vi "Lockin.getDAQPublicEvents.vi"(8 "error in (no error)":errorcluster, 11 "Instrument.Lockin in":refnum<class "Instrument.Lockin.lvclass">) -> (0 "error out":errorcluster, 1 "DAQ SMO Public Events":T2, 2 "DAQ Public Events":T1, 3 "Instrument.Lockin out":refnum<class "Instrument.Lockin.lvclass">)   [LabVIEW 2019, in "Instrument.Lockin.lvlib" / "Instrument.Lockin.lvclass"]
uses:
  Instrument.Lockin.lvclass
  <vilib>/JKI/JKI SMO/SMO/Typedefs/Public Events.ctl
  <vilib>/JKI/JKI SMO/SMO/Typedefs/SMOState --Enum.ctl
  <vilib>/JKI/JKI SMO/SMO/Typedefs/Reserve State--Enum.ctl
  Instrument.DAQ/Typedefs/PublicEvents--Cluster.ctl
  Instrument.DAQ/Typedefs/PublicEvents--DAQ.getAIChannels.ctl
  Instrument.DAQ/Typedefs/AI.Channel--Cluster--Array.ctl
  Instrument.DAQ/Typedefs/AI.Channel--Cluster.ctl
  Instrument.DAQ/Typedefs/PublicEvents--DAQ.getAOChannels.ctl
  Instrument.DAQ/Typedefs/AO.Channel--Cluster--Array.ctl
  Instrument.DAQ/Typedefs/AO.Channel--Cluster.ctl
  Instrument.DAQ/Typedefs/AO.Channel.Function--Enum.ctl
  Instrument.DAQ/Typedefs/PublicEvents--DAQ.getREFChannels.ctl
  Instrument.DAQ/Typedefs/REF.Channel--Cluster--Array.ctl
  Instrument.DAQ/Typedefs/REF.Channel--Cluster.ctl
  Instrument.DAQ/Typedefs/PublicEvents--DAQ.getWaveforms.ctl
  Instrument.DAQ/Typedefs/PublicEvents--DAQ.getResults.ctl
  Instrument.DAQ/Typedefs/Results--Cluster.ctl
  Instrument.DAQ/Typedefs/PublicEvents--DAQ.getSweepWaveforms.ctl
  Instrument.DAQ/Typedefs/PublicEvents--DAQ.getCalibration.ctl
  Instrument.DAQ/Typedefs/DAQ.Calibration--Cluster--Array.ctl
  Instrument.DAQ/Typedefs/DAQ.Calibration--Cluster.ctl
  Instrument.DAQ/Typedefs/PublicEvents--DAQ.getDAQState.ctl
  Instrument.DAQ/Typedefs/Status--enum.ctl
  Instrument.DAQ/Typedefs/PublicEvents--DAQ.getDAQconfig.ctl
  Instrument.DAQ/Typedefs/DAQ.Configuration--Cluster--Array.ctl
  Instrument.DAQ/Typedefs/DAQ.Configuration--Cluster.ctl
  Instrument.DAQ/Typedefs/DAQ.Config.AO.Range--enum.ctl
  Instrument.DAQ/Typedefs/DAQ.TerminalConfiguration--ring.ctl
  Instrument.DAQ/Typedefs/DAQ.Config.AI.Range--enum.ctl
  Instrument.DAQ/Typedefs/DAQ.Config.AI.Coupling--enum.ctl
  Instrument.DAQ/Typedefs/PublicEvents--DAQ.getInputGain.ctl
  Instrument.DAQ/Typedefs/Channel.Gain--Cluster--Array.ctl
  Instrument.DAQ/Typedefs/Channel.Gain--Cluster.ctl
  Instrument.DAQ/Typedefs/PublicEvents--DAQ.getOutputGain.ctl
  Instrument.DAQ/Typedefs/PublicEvents--DAQ.getInputOffset.ctl
  Instrument.DAQ/Typedefs/PublicEvents--DAQ.getSampling.ctl
  Instrument.DAQ/Typedefs/DAQ.Sampling--Cluster.ctl
  Instrument.DAQ/Typedefs/DAQ.Sampling.Sampling--Cluster.ctl
  Instrument.DAQ/Typedefs/DAQ.Sampling.Fs Mode--enum.ctl
  Instrument.DAQ/Typedefs/PublicEvents--DAQ.getSweepChannels.ctl
  Instrument.DAQ/Typedefs/Sweep.Configuration--Cluster.ctl
  Instrument.DAQ/Typedefs/Sweep.Channel--Cluster--Array.ctl
  Instrument.DAQ/Typedefs/Sweep.Channel--Cluster.ctl
  Instrument.DAQ/Typedefs/Sweep.Pattern--Enum.ctl
  Instrument.DAQ/Typedefs/PublicEvents--DAQ.getDeviceIDN.ctl
  Instrument.DAQ/Typedefs/DeviceInfo--Cluster.ctl
  <vilib>/JKI/JKI SMO/SMO/SMO.lvclass/SMO.ctl
  <vilib>/JKI/JKI SMO/SMO/Private/ReftoDVR--SMO.vi
  Instrument.DAQ/Instrument.DAQ.lvclass
  C:/Program Files/National Instruments/LabVIEW 2019/vi.lib/JKI/JKI SMO/SMO/SMO.lvclass
  <vilib>/JKI/JKI SMO/SMO/SMO.lvclass
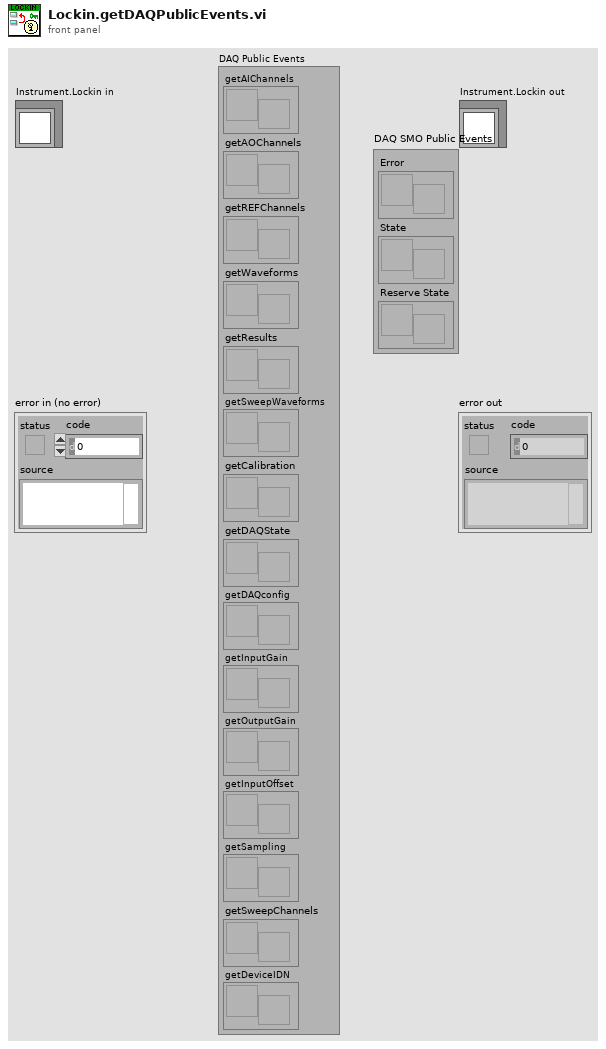
[diagram p1: front panel]
types:
  T1 = typedef "Instrument.Lockin.lvlib/Instrument.DAQ.lvclass/PublicEvents--Cluster.ctl" = cluster{"getAIChannels":refnum<user-event>, "getAOChannels":refnum<user-event>, "getREFChannels":refnum<user-event>, "getWaveforms":refnum<user-event>, "getResults":refnum<user-event>, "getSweepWaveforms":refnum<user-event>, "getCalibration":refnum<user-event>, "getDAQState":refnum<user-event>, "getDAQconfig":refnum<user-event>, "getInputGain":refnum<user-event>, "getOutputGain":refnum<user-event>, "getInputOffset":refnum<user-event>, "getSampling":refnum<user-event>, "getSweepChannels":refnum<user-event>, "getDeviceIDN":refnum<user-event>}
  T2 = typedef "SMO.lvclass/Public Events.ctl" = cluster{"Error":refnum<user-event>, "State":refnum<user-event>, "Reserve State":refnum<user-event>}
  T3 = typedef "Instrument.Lockin.lvlib/Instrument.Lockin.lvclass/Lockin.Dependencies--Cluster.ctl" = cluster{"Instrument.DAQ":refnum<class "Instrument.DAQ.lvclass">}
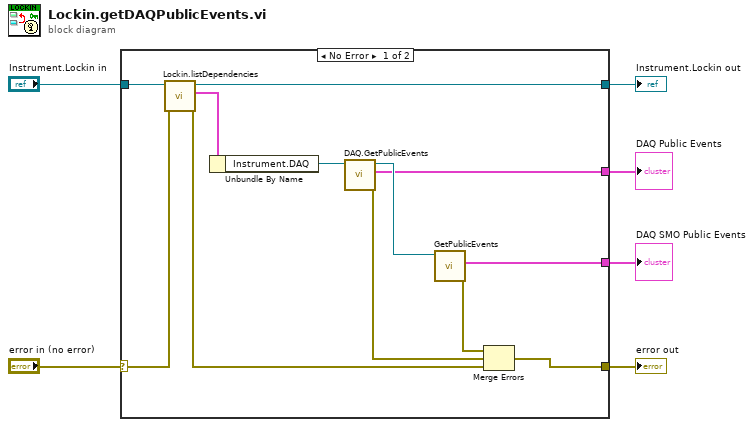
[diagram p0: block diagram]
diagram:
  n1 = case shown="No Error" "error in (no error)" {
    selector: "error in (no error)" -> [w10 w19]
    tunnel: [w13 w19] -> w5
    tunnel: [w9 w20] -> w3
    tunnel: "Instrument.Lockin in" -> [w12 w20]
    tunnel: [w17 _] -> w2
    tunnel: [w16 _] -> w1
    frame No Error {
      n2 = call "Lockin.listDependencies.vi"("error in (no error)"=w10, "Instrument.Lockin in"=w12) -> ("error out"=w11:errorcluster, "Dependencies"=w8:T3, "Instrument.Lockin out"=w9:refnum<class "Instrument.Lockin.lvclass">)  [unwired: 7 in]
      n3 = Unbundle By Name(w8) -> ("Instrument.DAQ"=w7:refnum<class "Instrument.DAQ.lvclass">)
      n4 = call "DAQ.GetPublicEvents.vi"("Instrument.DAQ"=w7) -> ("error out"=w14:errorcluster, "DAQ Public Events"=w16:T1, "Instrument.DAQ out"=w18:refnum<class "Instrument.DAQ.lvclass">)  [unwired: 8 in]
      n5 = call <vilib>:"GetPublicEvents.vi"("SMO"=w18) -> ("error out"=w15:errorcluster, "Public Events"=w17:T2)  [unwired: 8 in, 1 out]
      n6 = Merge Errors(w15, w14, w11) -> (w13:errorcluster)
    }
    frame Error {
    }
  }
  "error out" <- w5
  "Instrument.Lockin out" <- w3
  "DAQ SMO Public Events" <- w2
  "DAQ Public Events" <- w1
